vi "LEIN CMD read ACTI.vi"(7 "CMD":T1={"SID"=0, "ANF"=FALSE, "CMD"=enum."TASK", "DATA"=[]}, 11 "error in (no error)":errorcluster) -> (4 "SID":u8, 6 "Data":u8[](array[numeric]), 8 "ACI ID":u8, 14 "ACK":bool, 15 "error out":errorcluster)   [LabVIEW 2011]
uses:
  Defenitions/LEIN CMD Cluster.ctl
  Defenitions/LEIN CMD List.ctl
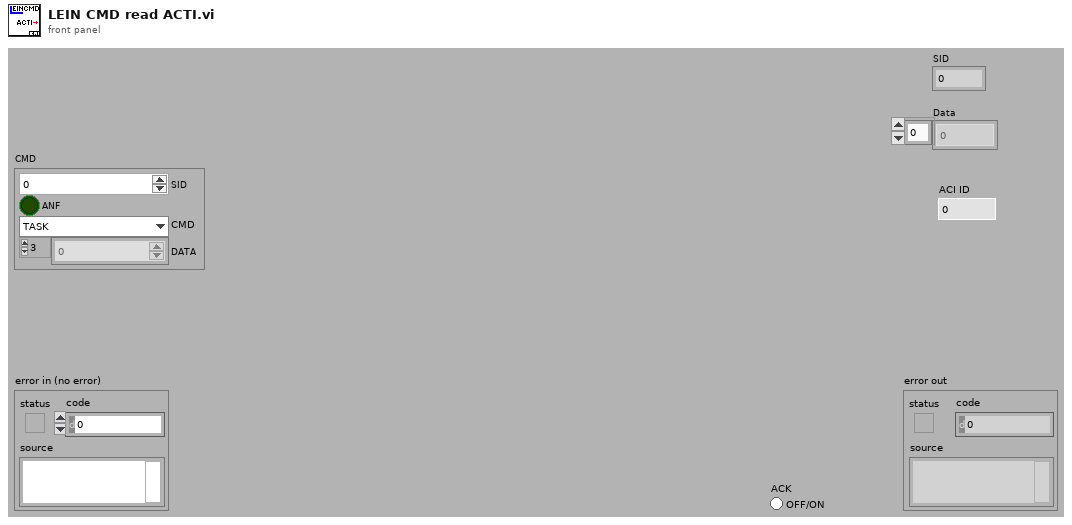
[diagram p1: front panel]
types:
  T1 = typedef "LEIN CMD Cluster.ctl" = cluster{"SID":u8, "ANF":bool, "CMD":T2, "DATA":u8[]}
  T2 = typedef "LEIN CMD List.ctl" = enum8{"ACTI", "TASK", "RES0", "STAT", "RES1", "RES2", "RES3", "USER"}
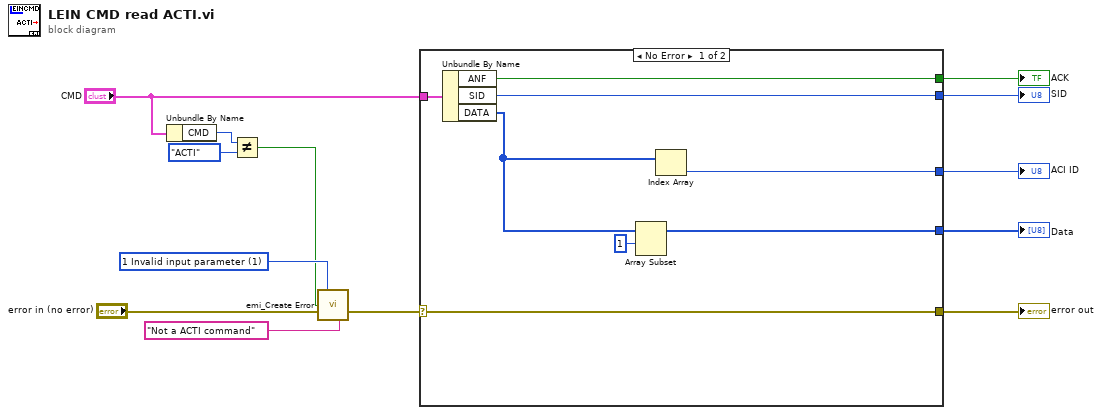
[diagram p0: block diagram]
diagram:
  w13 = 1 items=["0 No Error"=0, "1 Invalid input parameter"=1, "6 Generic file IO "=6, "7 File not Found"=7, "35 Generic Pring Error"=35, "37 Device not Found"=37, "39 Device Unit Error"=39, "40 Could fot Open Device"=40, "42 Generic Error"=42, "52 Unknown Message"=52, "98 Bad File type"=98, "99 Bad File Version"=99, "100 Bad Data in File"=100, "1018 Unspecefied Error"=1018, "1041 Incorrect Password"=1041, "1043 Feature not in this version"=1043, "1109 Unsuported Data type"=1109, "1444 Did not close sucessfully"=1444] ("Error Code")
  n1 = Unbundle By Name("CMD") -> ("CMD"=w8:T2)
  n2 = Not Equal?(x=w8, y=LEIN_CMD_List."ACTI") -> (x != y?=w6:bool)
  n3 = call "emi_Create Error.vi"("Error Code"=w13, "Error(T)"=w6, "error in (no error)"="error in (no error)", "Append String(\"\")"="Not a ACTI command" ("Append String(\"\")")) -> ("error out"=w9:errorcluster)  [unwired: 11 in]
  n4 = case shown="No Error" w9 {
    selector: w9 -> [w18 w22]
    tunnel: [w18 w22] -> w10
    tunnel: "CMD" -> [w21 _]
    tunnel: [w20 _] -> w4
    tunnel: [w19 _] -> w3
    tunnel: [w16 _] -> w2
    tunnel: [w14 _] -> w1
    frame No Error {
      n5 = Unbundle By Name(w21) -> ("ANF"=w19:bool, "SID"=w20:u8, "DATA"=w17:u8[])
      n6 = Array Subset(array=w17, index=1) -> (w16:u8[])  [unwired: 1 in]
      n7 = Index Array(array=w17) -> (element=w14:u8)  [unwired: 1 in]
    }
    frame Error {
    }
  }
  "error out" <- w10
  "SID" <- w4
  "ACK" <- w3
  "Data" <- w2
  "ACI ID" <- w1
